vi "open server method.vi"(7 "DS method in":T1={"scan rate (Hz)"=100.0, "Channel group array"=[], "Number of groups"=1} {"Number of groups" min=1; "Channel group array"."max voltage" format="%.4f"; "scan rate (Hz)" format="%.2f"}) -> (0 "DS method":T1={"scan rate (Hz)"=100.0, "Channel group array"=[], "Number of groups"=1} {"Number of groups" min=1; "Channel group array"."max voltage" format="%.4f"; "scan rate (Hz)" format="%.2f"}, 3 "canceled":bool)   [LabVIEW 2012]
uses:
  DataServer/Dataserver method.ctl
panel:
  # "Hz"
  # "channel identifiers"
  # "max voltage"
  # "port locations"
  # "Hz"
  # "channel identifiers"
  # "max voltage"
  # "port locations"
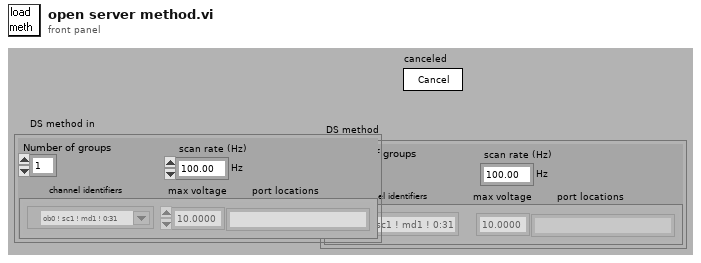
[diagram p1: front panel]
types:
  T1 = typedef "Dataserver method.ctl" = cluster{"scan rate (Hz)":dbl, "Channel group array":cluster{"channels":tag, "max voltage":sgl, "Port locations":string}[], "Number of groups":u8}
  T2 = enum16{"open", "open or create", "create or replace", "create", "open (read only)"}
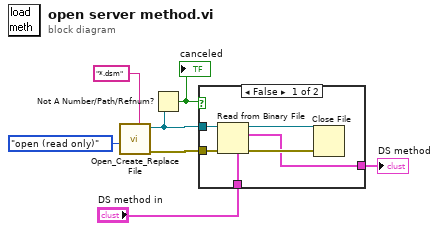
[diagram p0: block diagram]
diagram:
  n1 = call <vilib>:"Open_Create_Replace File.vi"("pattern"="*.dsm", "function (open:0)"=T2."open (read only)") -> ("error out"=w7:errorcluster, "refnum"=w2:refnum<file>)  [unwired: 6 in, 2 out]
  n2 = Not A Number/Path/Refnum?(number/path/refnum=w2) -> (NaN/Path/Refnum?=w1:bool)
  "canceled" <- w1
  n3 = case shown="False" w1 {
    tunnel: w7 -> [w13 _]
    tunnel: w2 -> [w12 _]
    tunnel: "DS method in" -> [w9 w14]
    tunnel: [w8 w14] -> w3
    frame False {
      n4 = Read from Binary File(5:w9, 8:w13, 11:w12) -> (0:w10:errorcluster, 2:w8:T1, 3:w11:refnum<file>)  [unwired: 3 in, 1 out]
      n5 = Close File(refnum=w11, error in=w10) -> ()  [unwired: 2 out]
    }
    frame True {
    }
  }
  "DS method" <- w3
